vi "solar_voy_def Quotes Add.vi"(10 "Whitespace Only? (F=Always)":bool, 11 "String":string) -> (3 "String with Comments":string)   [LabVIEW 2018]
doc: "This adds quotes to the string."
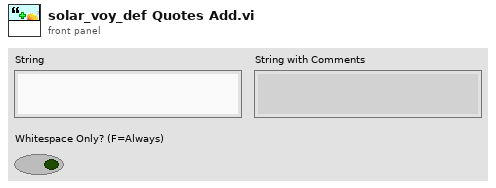
[diagram p1: front panel]
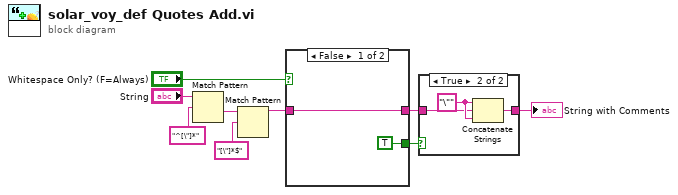
[diagram p0: block diagram]
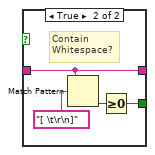
[diagram p2: hidden frame]
diagram:
  n1 = Match Pattern(string="String", regular expression="^[\"]*") -> (after substring=w8:string)  [unwired: 1 in, 3 out]
  n2 = Match Pattern(string=w8, regular expression="[\"]*$") -> (before substring=w5:string)  [unwired: 1 in, 3 out]
  n3 = case shown="False" "Whitespace Only? (F=Always)" {
    tunnel: w5 -> [w11 w12]
    tunnel: [TRUE w13] -> w3
    tunnel: [w11 w12] -> w1
    frame False {
    }
    frame True {
      # "Contain\nWhitespace?"
      n4 = Match Pattern(string=w12, regular expression="[ \t\r\n]") -> (offset past match=w14:i32)  [unwired: 1 in, 3 out]
      n5 = Greater Or Equal To 0?(x=w14) -> (x >= 0?=w13:bool)
    }
  }
  n6 = case shown="True" w3 {
    tunnel: w1 -> [w16 w18]
    tunnel: [w16 w17] -> w4
    frame False {
    }
    frame True {
      w19 = "\"" ("string")
      n7 = Concatenate Strings(w19, w18, w19) -> (w17:string)
    }
  }
  "String with Comments" <- w4
